vi "AES-Cipher-BLOCK.vi"(8 "error in (no error)":errorcluster, 10 "Cipher Key":u8[](array[numeric]) format="%02x", 11 "Plain [U8]":u8[](array[numeric]) format="%02x") -> (0 "error out":errorcluster, 3 "cipher [U8]":u8[](array[numeric]) format="%02x")   [LabVIEW 2011, in "i3-external-encryption.lvlib"]
doc: "Encripts the U8 block (16 bytes) using AES with the given cipher.\n\nCAUTION:\nThis VI is not secure, it does not protect the memory of the encryption, key and unencrypted data.\n\n(c) Ton Plomp, 2011\nTHIS SOFTWARE IS PROVIDED AS IS, AND ANY WARRANTY IS REJECTED"
uses:
  i3-external-encryption.lvlib
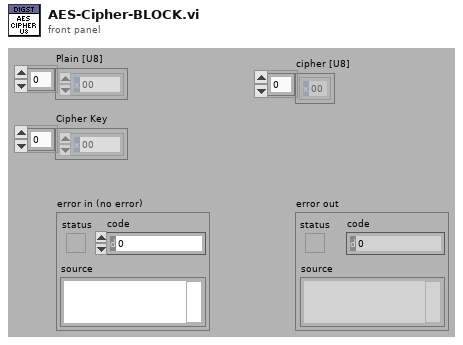
[diagram p1: front panel]
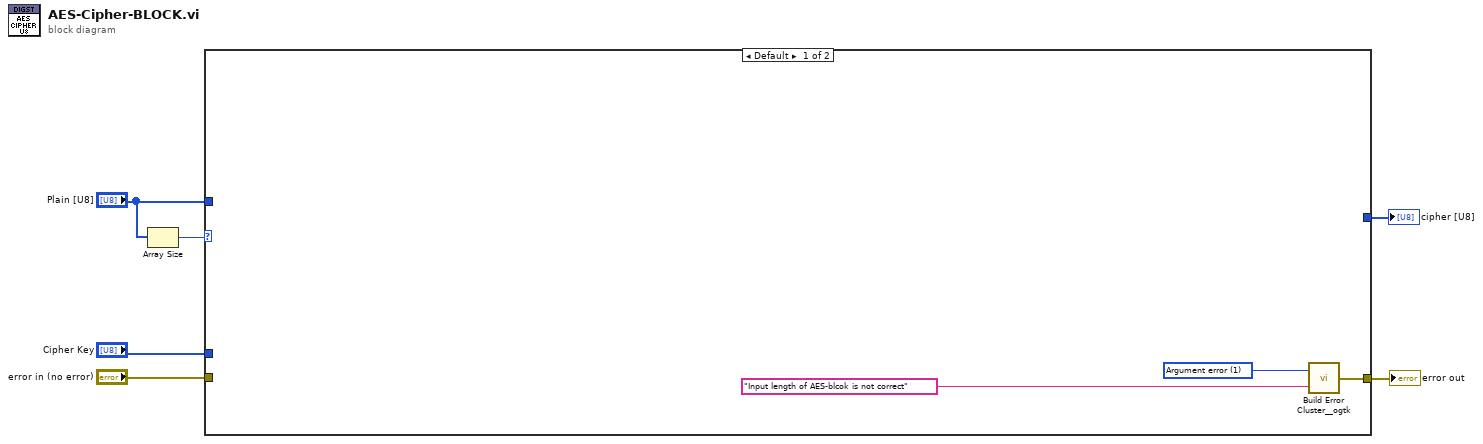
[diagram p0: block diagram]
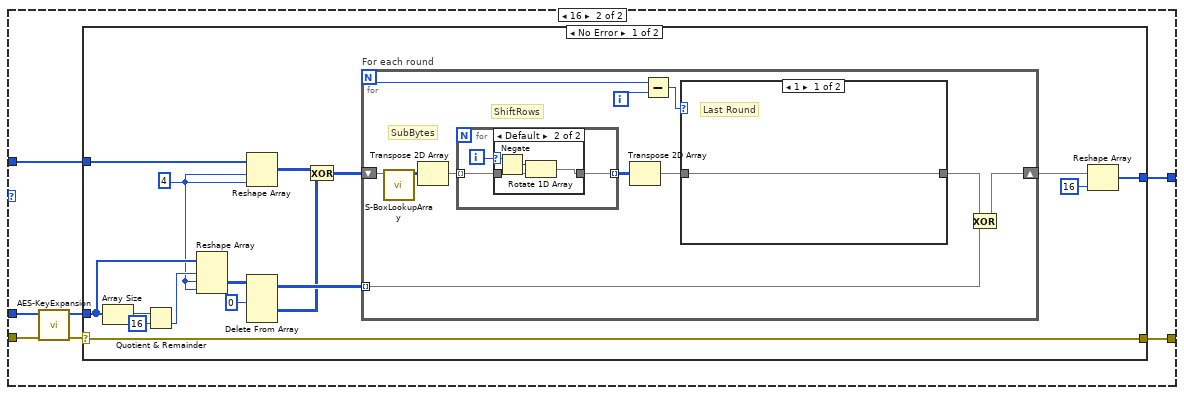
[diagram p2: hidden frame]
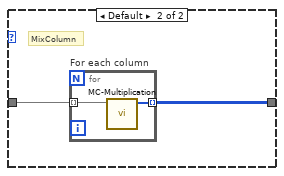
[diagram p3: hidden frame]
diagram:
  n1 = Array Size(array="Plain [U8]") -> (size(s)=w2:i32)
  n2 = case shown="Default" w2 {
    tunnel: [_ w15] -> w6
    tunnel: "Cipher Key" -> [_ w14]
    tunnel: "error in (no error)" -> [_ w13]
    tunnel: "Plain [U8]" -> [_ w12]
    tunnel: [w9 w10] -> w1
    frame Default {
      w8 = 1 items=["No error", "Argument error", "Memory is full", "Out of zone", "End of file", "File already open", "Generic file I/O error", "File not found", "File permission error", "Disk is full", "Duplicate path", "Too many files open", "System feature not enabled", "Resource file not found", "Cannot add resource", "Resource not found", "Image not found", "Image memory error", "Pen does not exist", "Config type invalid", "Config token not found", "Config parse error", "Config memory error", "Bad external code format", "Bad external code offset", "External code not present", "Null window", "Destroy window error", "Null menu", "Print aborted", "Bad print record", "Print driver error", "Windows error during printing", "Memory error during printing", "Print dialog error", "Generic print error", "Invalid device refnum", "Device not found", "Device parameter error", "Device unit error", "Cannot open device", "Device call aborted", "Generic error", "Cancelled by user", "Object ID too low", "Object ID too high", "Object not in heap", "Unknown heap", "Unknown object (invalid DefProc)", "Unknown object (DefProc not in table)", "Message out of range", "Invalid (null) method", "Unknown message", "Manager call not supported", "Bad address", "Network operation in progress", "Network operation timed out", "Connection is busy", "Network attribute not supported", "Network error", "Address in use", "System out of memory", "Connection aborted", "Connection refused", "Not connected", "Already connected", "Connection closed", "Initialization error (interapplication manager)", "Bad occurrence", "Wait on unbound occurrence handler", "Occurrence queue overflow", "Datalog type conflict", "Unused", "Unrecognized type (interapplication manager)", "Memory corrupt", "Failed to make temporary DLL", "Old CIN version", "Drag socket not found", "Failed to load drop-object", "Failed to register OLE object", "Failed to release OLE object", "Format specifier type mismatch", "Unknown format specifier", "Too few format specifiers", "Too many format specifiers", "Scan failed", "Newer CIN version", "Error converting to variant", "Runtime menu error", "Password tampered", "Variant attribute not found", "Incompatible variant data type", "Event data is not available", "Event Store is not present", "Occurrence is not found", "Event Queue is not created", "Event info is not available", "Refnum passed is NULL", "Error retrieving Class GUID", "Error retrieving CoClass GUID", "Error retrieving TypeLib GUID.", "Bad built application magic bytes.", "Specific driver is different from the specific driver associated with the Logical Name.", "There is no session opened to the class driver.", "Max Error", "MAX - Error with config objects", "MAX - Error loading configuration", "MAX - Group not supported"]
      n3 = call <userlib>:"Build Error Cluster__ogtk.vi"("String to Prepend to source (\"\")"="Input length of AES-blcok is not correct" ("String to Prepend to source (\"\")"), "code"=w8) -> ("error out"=w9:errorcluster)
    }
    frame 16 {
      n4 = call "AES-KeyExpansion.vi"("error in (no error)"=w13, "Key In"=w14) -> ("error out"=w11:errorcluster, "Expanded Key [U8]"=w16:u8[])  [unwired: 8 in]
      n5 = case shown="No Error" w11 {
        selector: w11 -> [w20 w57]
        tunnel: w16 -> [w30 _]
        tunnel: [w24 _] -> w15
        tunnel: w12 -> [w22 _]
        tunnel: [w20 w57] -> w10
        frame No Error {
          w21 = 4 ("y")
          n6 = Array Size(array=w30) -> (size(s)=w32:i32)
          n7 = Quotient & Remainder(x=w32, y=16) -> (floor(x/y)=w27:i32)  [unwired: 1 out]
          n8 = Reshape Array(w30, w27, w21, w21) -> (w17:u8[][][])
          n9 = Reshape Array(w22, w21, w21) -> (w19:u8[][])
          n10 = Delete From Array(array=w17, index (dim 0)=0 ("disabled index (col)")) -> (deleted portion=w18:u8[][], array with subset deleted=w29:u8[][][])  [unwired: 3 in]
          n11 = Exclusive Or(1:w18, 2:w19) -> (0:w28:u8[][])
          n12 = for "For each round" {
            N -> [w41]
            shift-right: [w37] -> w25
            shift-left: w28 -> [w43]
            tunnel: w29 -> [w38] mode=indexing
            i -> [w40]
            # "ShiftRows"
            # "SubBytes"
            n13 = call "S-BoxLookupArray.vi"("In"=w43) -> ("Out"=w36:u8[][])  [unwired: 10 in]
            n14 = Transpose 2D Array(2D array=w36) -> (transposed array=w34:u8[][])
            n15 = for {
              tunnel: w34 -> [w50] mode=indexing
              tunnel: [w49] -> w35 mode=indexing
              i -> [w51]
              n16 = case shown="Default" w51 {
                selector: w51 -> [_ w55]
                tunnel: w50 -> [w52 w56]
                tunnel: [w52 w54] -> w49
                frame 0 {
                }
                frame Default {
                  n17 = Negate(x=w55) -> (-x=w53:i32)
                  n18 = Rotate 1D Array(1:w56, 2:w53) -> (0:w54:u8[])
                }
              }
            }
            n19 = Transpose 2D Array(2D array=w35) -> (transposed array=w33:u8[][])
            n20 = Subtract(x=w41, y=w40) -> (x-y=w39:i32)
            n21 = case shown="1" w39 {
              tunnel: w33 -> [w44 w46]
              tunnel: [w44 w45] -> w42
              frame 1 {
                # "Last Round"
              }
              frame Default {
                # "MixColumn"
                n22 = for "For each column" {
                  tunnel: w46 -> [w47] mode=indexing
                  tunnel: [w48] -> w45 mode=indexing
                  n23 = call "MC-Multiplication.vi"("Vector In"=w47) -> ("Vector Out"=w48:u8[])  [unwired: 10 in]
                }
              }
            }
            n24 = Exclusive Or(1:w38, 2:w42) -> (0:w37:u8[][])
          }
          n25 = Reshape Array(w25, 16 ("dimension size")) -> (w24:u8[])
        }
        frame Error {
        }
      }
    }
  }
  "error out" <- w1
  "cipher [U8]" <- w6
